vi "Read_Data.vi"(8 "error in":errorcluster caption="entrée d'erreur") -> (0 "error out":errorcluster caption="sortie d'erreur", 1 "AO Slave":waveform(dbl)[](array[waveform]), 2 "AO Master":waveform(dbl)[](array[waveform]), 3 "DO Master":digitalwaveform[](graph))   [LabVIEW 2026]
panel:
  out "Tableau":digitalwaveform[](array[waveform])
  out "nom des voies en sortie 3":string[](array[string])
  out "nom des voies en sortie 2":string[](array[string])
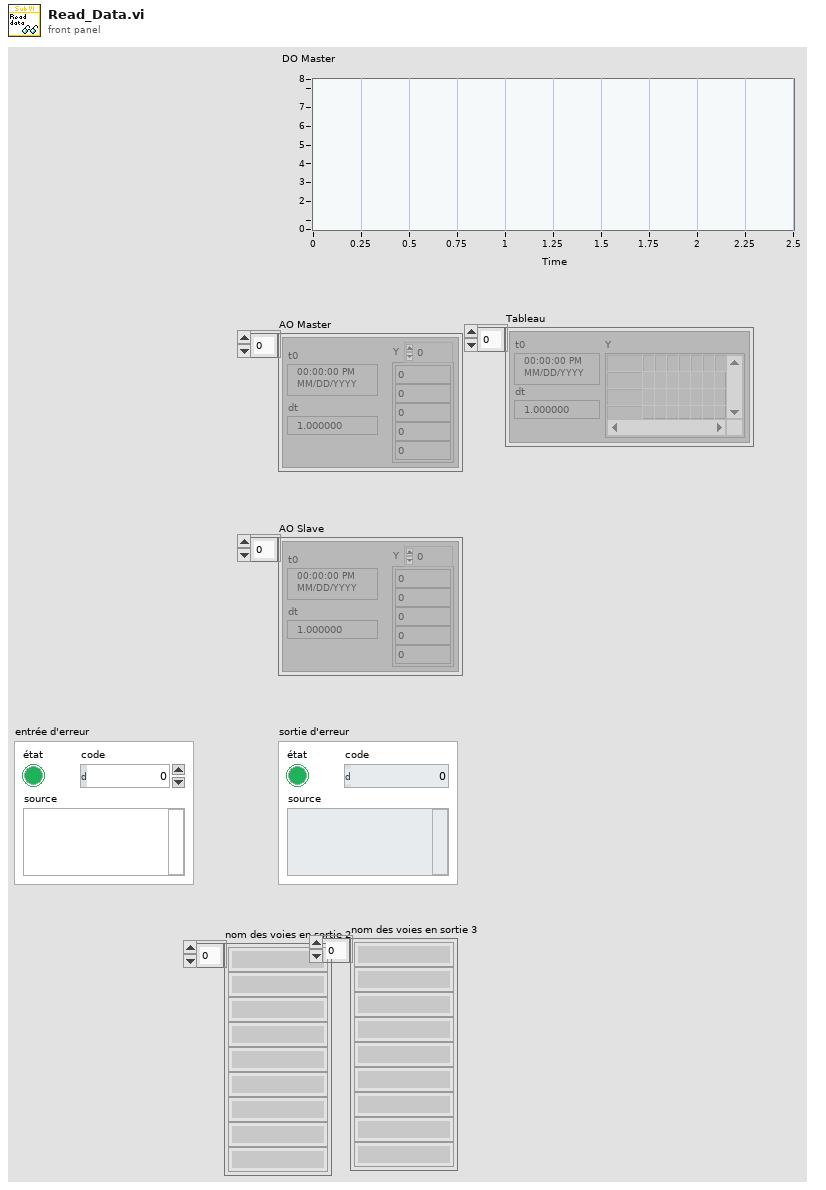
[diagram p1: front panel]
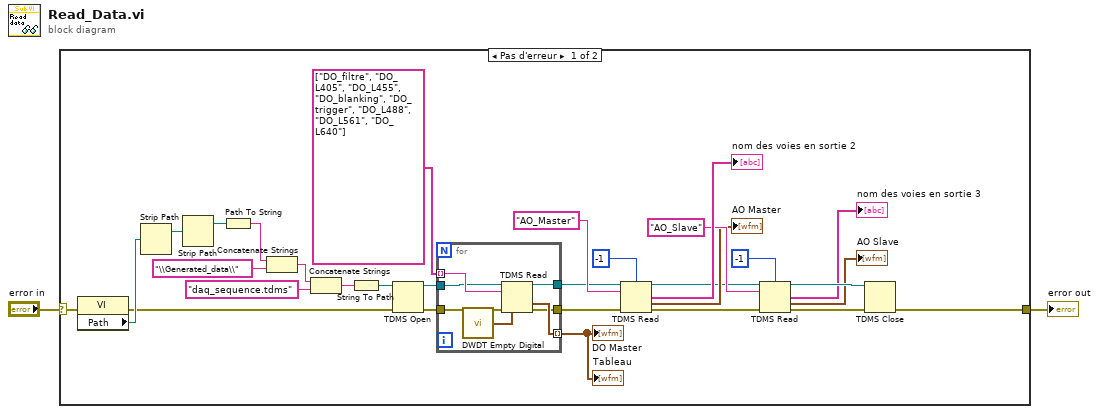
[diagram p0: block diagram]
diagram:
  n1 = case shown="Pas d'erreur" "error in" {
    selector: "error in" -> [w25 w40]
    tunnel: [w13 w40] -> w1
    frame No Error {
      n2 = property class="VI"(error in=w25) -> (error out=w9:errorcluster, "Path"=w31:path)  [unwired: 1 in, 1 out]
      n3 = Strip Path(path=w31) -> (stripped path=w30:path)  [unwired: 1 out]
      n4 = Strip Path(path=w30) -> (stripped path=w29:path)  [unwired: 1 out]
      n5 = Path To String(path=w29) -> (string=w32:string)
      n6 = Concatenate Strings(w32, "\\Generated_data\\" ("Python_file")) -> (w26:string)
      n7 = Concatenate Strings(w26, "daq_sequence.tdms" ("File_to_read")) -> (w24:string)
      n8 = String To Path(string=w24) -> (path=w20:path)
      n9 = TDMS Open(8:w9, 11:w20) -> (0:w7:errorcluster, 3:w4:refnum<k34>)  [unwired: 5 in]
      n10 = for {
        tunnel: string[] ["DO_filtre", "DO_L405", "DO_L455", "DO_blanking", "DO_trigger", "DO_L488", "DO_L561", "DO_L640"] ("nom des voies en sortie") -> [w37] mode=indexing
        tunnel: [w39] -> w5 mode=indexing
        tunnel: w7 -> [w36]
        tunnel: [w35] -> w6
        tunnel: w4 -> [w34]
        tunnel: [w33] -> w3
        n11 = call <vilib>:"DWDT Empty Digital.vi"() -> ("digital waveform out"=w38:digitalwaveform)  [unwired: 5 in]
        n12 = TDMS Read(0:w34, 5:w37, 11:w36, 12:w38) -> (4:w33:refnum<k34>, 10:w39:digitalwaveform, 15:w35:errorcluster)  [unwired: 4 in, 3 out]
      }
      "DO Master" <- w5
      "Tableau" <- w5
      n13 = TDMS Read(0:w3, 2:i64 -1 ("nombre (-1: tous)"), 5:"AO_Master" ("nom du groupe en entrée"), 11:w6) -> (4:w10:refnum<k34>, 8:→"nom des voies en sortie 2":string[], 10:→"AO Master":waveform(dbl)[], 15:w11:errorcluster)  [unwired: 4 in, 2 out]
      n14 = TDMS Read(0:w10, 2:i64 -1 ("nombre (-1: tous)"), 5:"AO_Slave" ("nom du groupe en entrée"), 11:w11) -> (4:w19:refnum<k34>, 8:→"nom des voies en sortie 3":string[], 10:→"AO Slave":waveform(dbl)[], 15:w18:errorcluster)  [unwired: 4 in, 2 out]
      n15 = TDMS Close(8:w18, 11:w19) -> (0:w13:errorcluster)  [unwired: 1 out]
    }
    frame Error {
    }
  }
  "error out" <- w1
